vi "Write Command.vi"(7 "Command":T1, 8 "error in (no error)":errorcluster, 9 "Value (0)":u8 format="%.0x", 10 "Session In":refnum<class "Session.lvclass">, 11 "PCF8574 I2C LCD in":refnum<class "PCF8574 I2C LCD.lvclass">) -> (0 "error out":errorcluster, 2 "Session Out":refnum<class "Session.lvclass">, 3 "PCF8574 I2C LCD out":refnum<class "PCF8574 I2C LCD.lvclass">)   [LabVIEW 2020, in "CTI-Peripheral.lvlib" / "PCF8574 I2C LCD.lvclass"]
uses:
  PCF8574 I2C LCD.lvclass
  CTI/Session/Session.lvclass
  HD44780 LCD/Command.ctl
  HD44780 LCD/HD44780 LCD.lvlib
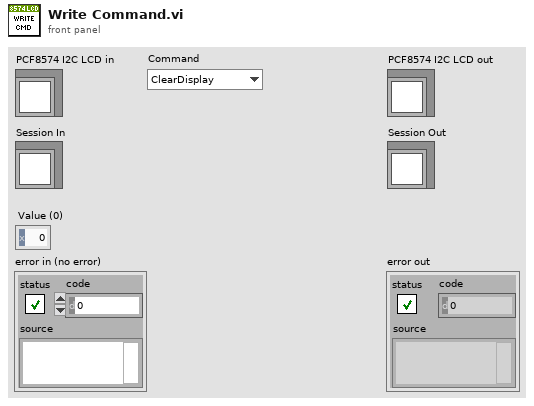
[diagram p1: front panel]
types:
  T1 = typedef "CTI-Peripheral.lvlib/HD44780 LCD.lvlib/Command.ctl" = enum16{"ClearDisplay", "ReturnHome", "EntryModeSet", "DisplayControl", "CursorShift", "FunctionSet", "SetCGRamAddr", "SetDDRamAddr"}
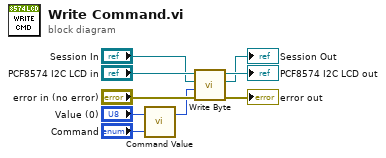
[diagram p0: block diagram]
diagram:
  n1 = call "Command Value.vi"("Value"="Value (0)", "Command"="Command") -> ("Byte"=w3:u8)  [unwired: 5 in]
  n2 = call "Write Byte.vi"("error in (no error)"="error in (no error)", "Value"=w3, "Session in"="Session In", "PCF8574 I2C LCD in"="PCF8574 I2C LCD in") -> ("error out"=→"error out":errorcluster, "Session out"=→"Session Out":refnum<class "Session.lvclass">, "PCF8574 I2C LCD out"=→"PCF8574 I2C LCD out":refnum<class "PCF8574 I2C LCD.lvclass">)  [unwired: 5 in]
